vi "UpdateDisplay.vi"(7 "error in (no error)":errorcluster, 8 "Gauge":refnum<vi>, 9 "Container State":T2, 10 "Display State In":T1) -> (0 "error out":errorcluster)   [LabVIEW 2012, in "CustomGauge.xctl"]
uses:
  CustomGauge.xctl
  <vilib>/_xctls/Container State.ctl
  CustomGaugeState.ctl
  <resource>/objmgr/nvio.rc
  <vilib>/_xctls/XControlSupport.lvlib
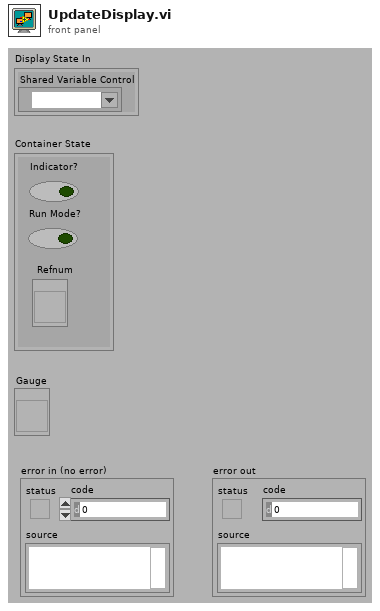
[diagram p1: front panel]
types:
  T1 = typedef "CustomGauge.xctl/CustomGaugeState.ctl" = cluster{"Shared Variable Control":refnum<k21>}
  T2 = typedef "XControlSupport.lvlib/Container State.ctl" = cluster{"Indicator?":bool, "Run Mode?":bool, " Refnum":refnum<vi>}
  T3 = enum32{"No PSP", "Read", "Write", "Write & Read"}
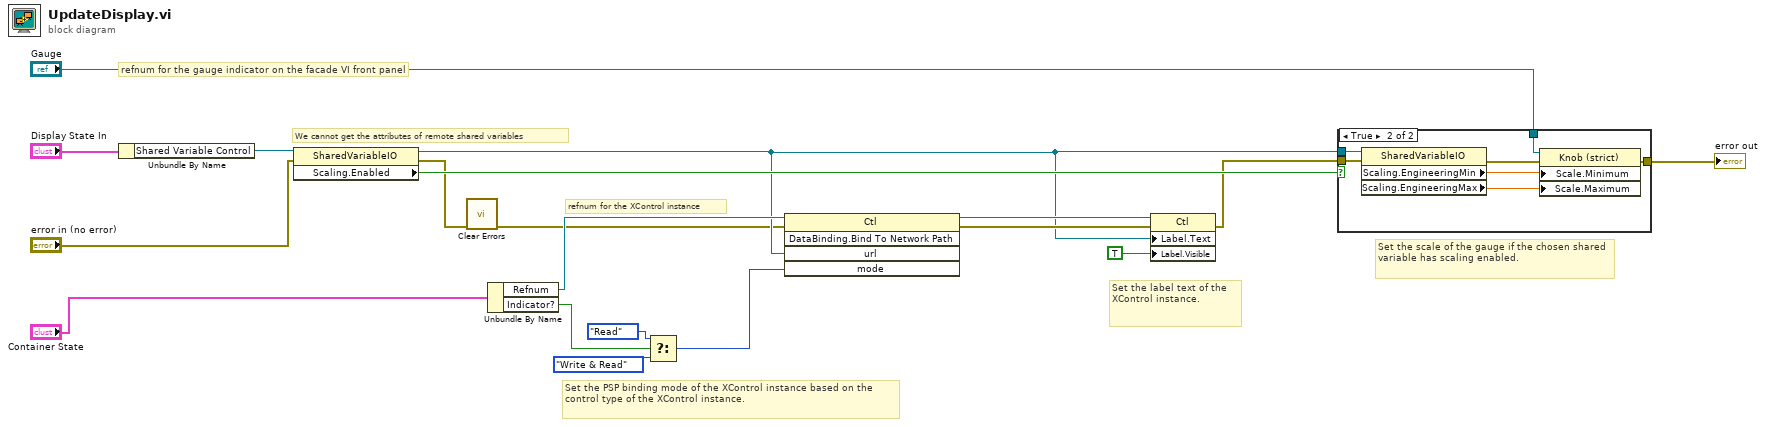
[diagram p0: block diagram]
diagram:
  # "We cannot get the attributes of remote shared variables"
  # "Set the scale of the gauge if the chosen shared variable has scaling enabled."
  # "refnum for the gauge indicator on the facade VI front panel"
  # "refnum for the XControl instance"
  # "Set the label text of the XControl instance."
  # "Set the PSP binding mode of the XControl instance based on the control type of the XControl instance."
  n1 = Unbundle By Name("Display State In") -> ("Shared Variable Control"=w3:refnum<k21>)
  n2 = property class="SharedVariableIO"(reference=w3, error in="error in (no error)") -> (reference out=w2:refnum<k21>, error out=w4:errorcluster, "Scaling.Enabled"=w18:bool)
  n3 = call <vilib>:"Clear Errors.vi"("error in (no error)"=w4) -> ("error out"=w1:errorcluster)  [unwired: 6 in]
  n4 = Unbundle By Name("Container State") -> ("Refnum"=w9:refnum<vi>, "Indicator?"=w16:bool)
  n5 = Select(t=T3."Read" ("Mode"), s=w16, f=T3."Write & Read" ("Mode")) -> (s? t:f=w13:T3)
  n6 = invoke class="Ctl" method="DataBinding.Bind To Network Path"(reference=w9, error in=w1, "url"=w2, "mode"=w13) -> (reference out=w10:refnum<vi>, error out=w6:errorcluster)  [unwired: 1 in, 3 out]
  n7 = property class="Ctl"(reference=w10, error in=w6, "Label.Text"=w2, "Label.Visible"=TRUE) -> (error out=w5:errorcluster)  [unwired: 1 out]
  n8 = case shown="True" w18 {
    tunnel: w2 -> [_ w27]
    tunnel: "Gauge" -> [_ w24]
    tunnel: w5 -> [w20 w23]
    tunnel: [w20 w21] -> w8
    frame False {
    }
    frame True {
      n9 = property class="SharedVariableIO"(reference=w27, error in=w23) -> (error out=w22:errorcluster, "Scaling.EngineeringMin"=w26:dbl, "Scaling.EngineeringMax"=w25:dbl)  [unwired: 1 out]
      n10 = property on="Property Node" class="Knob (strict)"(reference=w24, error in=w22, "Scale.Minimum"=w26, "Scale.Maximum"=w25) -> (error out=w21:errorcluster)  [unwired: 1 out]
    }
  }
  "error out" <- w8
